vi "SwerveMotorControl.vi"(6 "Numeric":dbl, 9 "Boolean":bool, 10 "Normalized Value":dbl) -> (1 "Out":dbl)   [LabVIEW 2014]
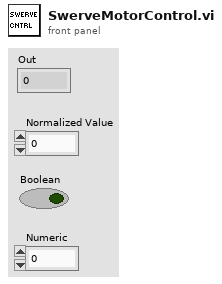
[diagram p1: front panel]
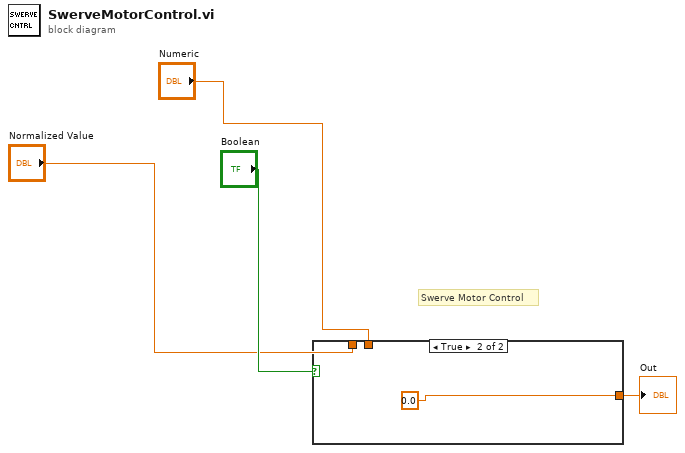
[diagram p0: block diagram]
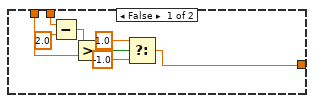
[diagram p2: hidden frame]
diagram:
  # "Swerve Motor Control"
  n1 = case shown="True" "Boolean" {
    tunnel: "Normalized Value" -> [w9 _]
    tunnel: "Numeric" -> [w11 _]
    tunnel: [w5 0.0 ("Motor Output")] -> w1
    frame False {
      n2 = Subtract(x=w11, y=2.0) -> (x-y=w10:dbl)
      n3 = Greater?(x=w10, y=w9) -> (0:w8:bool)
      n4 = Select(t=1.0, s=w8, f=-1.0) -> (s? t:f=w5:dbl)
    }
    frame True {
    }
  }
  "Out" <- w1
